vi "Read Register.vi"(5 "CS (None)":refnum<class "SPI CS.lvclass">, 6 "Read Delay ms (5)":u32=5, 7 "SPI":refnum<class "SPI.lvclass">, 8 "error in (no error)":errorcluster, 9 "Len":u8, 10 "Register":u8 format="%.0x", 11 "Session In":refnum<class "Session.lvclass">) -> (0 "error out":errorcluster, 1 "Data":string, 3 "Session Out":refnum<class "Session.lvclass">)   [LabVIEW 2024, in "CTI.lvlib" / "SPI.lvclass"]
uses:
  SPI.lvclass
  Session/Session.lvclass
  SPI CS/SPI CS.lvclass
  SPI.lvclass/SPI.ctl
  dd603ebe-05eb-4c36-9332-c4d71327013a.vi
  Session/SPI Write Data.vi
  Session/SPI Read Data.vi
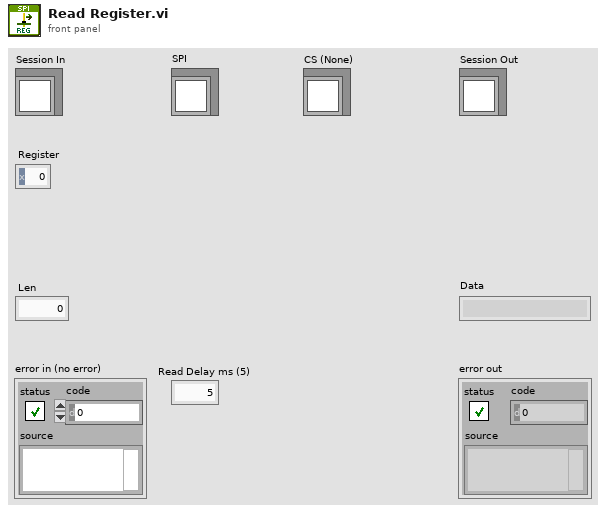
[diagram p1: front panel]
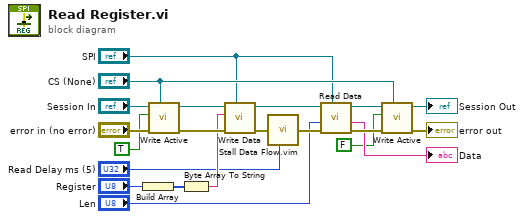
[diagram p0: block diagram]
diagram:
  n1 = Build Array("Register") -> (w14:u8[])
  n2 = call "Write Active.vi"("SPI CS"="CS (None)", "error in (no error)"="error in (no error)", "Active"=TRUE, "Session In"="Session In") -> ("error out"=w17:errorcluster, "Session Out"=w16:refnum<class "Session.lvclass">)  [unwired: 6 in]
  n3 = Byte Array To String(unsigned byte array=w14) -> (string=w13:string)
  n4 = call "Write Data.vi"("SPI"="SPI", "error in (no error)"=w17, "Data"=w13, "Session In"=w16) -> ("error out"=w11:errorcluster, "Session Out"=w12:refnum<class "Session.lvclass">)  [unwired: 6 in]
  n5 = call "Stall Data Flow.vim"("value in"=w11, "milliseconds to wait"="Read Delay ms (5)") -> ("value out"=w3:errorcluster)  [unwired: 1 out]
  n6 = call "Read Data.vi"("SPI"="SPI", "error in (no error)"=w3, "Len"="Len", "Session In"=w12) -> ("error out"=w21:errorcluster, "Data"=→"Data":string, "Session Out"=w9:refnum<class "Session.lvclass">)  [unwired: 5 in]
  n7 = call "Write Active.vi"("SPI CS"="CS (None)", "error in (no error)"=w21, "Active"=FALSE, "Session In"=w9) -> ("error out"=→"error out":errorcluster, "Session Out"=→"Session Out":refnum<class "Session.lvclass">)  [unwired: 6 in]
